vi "Get Version Information.vi"(8 "error in (no error)":errorcluster, 11 "Test Executive Builder Model in":refnum<class "Test Executive Builder Model.lvclass">) -> (0 "error out":errorcluster, 2 "Version Info":string, 3 "Test Executive Builder Model out":refnum<class "Test Executive Builder Model.lvclass">)   [LabVIEW 2017, in "Test Executive Builder Model.lvclass"]
uses:
  Test Executive Builder Model.lvclass
  <vilib>/gpm_packages/@cs/test-executive/Source/Test Executive/TestExecutive Ref/TestExecutive Ref.lvclass
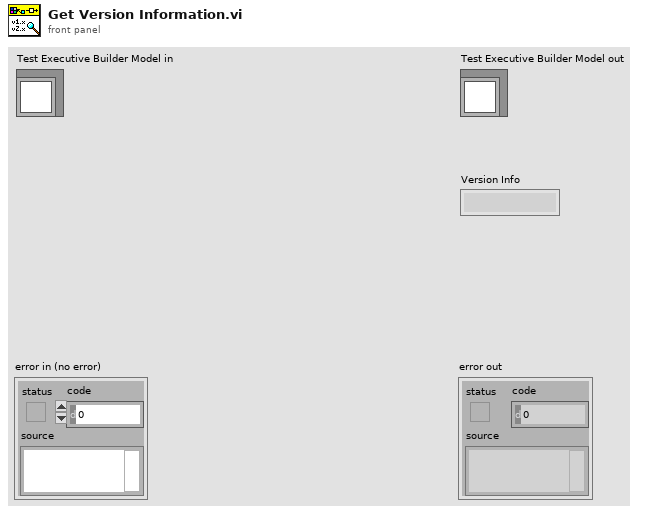
[diagram p1: front panel]
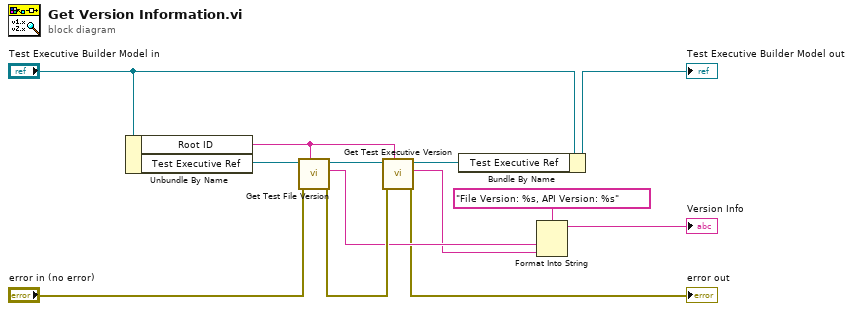
[diagram p0: block diagram]
diagram:
  n1 = Unbundle By Name("Test Executive Builder Model in") -> ("Root ID"=w5:string, "Test Executive Ref"=w6:refnum<data-value>)
  n2 = call <vilib>:"Get Test File Version.vi"("Unique ID"=w5, "error in (no error)"="error in (no error)", "Test Executive Ref"=w6) -> ("error out"=w12:errorcluster, "Test File Version"=w11:string, "Test Executive Ref out"=w13:refnum<data-value>)  [unwired: 5 in, 1 out]
  n3 = call <vilib>:"Get Test Executive Version.vi"("Unique ID"=w5, "error in (no error)"=w12, "Test Executive Ref"=w13) -> ("error out"=→"error out":errorcluster, "Test Executive Version"=w10:string, "Test Executive Ref out"=w4:refnum<data-value>)  [unwired: 5 in, 1 out]
  n4 = Bundle By Name(cluster="Test Executive Builder Model in", "Test Executive Ref"=w4) -> (→"Test Executive Builder Model out":refnum<class "Test Executive Builder Model.lvclass">)
  n5 = Format Into String(format string="File Version: %s, API Version: %s", w11, w10) -> (resulting string=→"Version Info":string)  [unwired: 2 in, 1 out]
